vi "rec_manipJumpDAQreplicates_v02.vi"(0 "AI task in":refnum<k21>, 1 "number of samples":i32=-1, 3 "controls array in":refnum<vi>[](array[refnum]), 4 "AO task in":refnum<k21>, 5 "error in":errorcluster, 6 "Start Position":T1(ring), 7 "Jump On Time (s)":dbl, 8 "Use Current Position for Start Pos?":bool, 9 "Duration (s)":dbl, 10 "Jump Position":T1(ring), 11 "Jump Duration (s)":dbl, 12 "common cluster":T2) -> (14 "AI task out":refnum<k21>, 15 "data out (pA or mV)":waveform(dbl)(graph), 17 "control array out":refnum<vi>[](array[refnum]), 18 "AO task out":refnum<k21>, 19 "error out":errorcluster)   [LabVIEW 2019]
uses:
  multipatch/controls/multipatch_common_controls_v4.ctl
  machine_vision/controls/transform_cluster_actuator.ctl
  machine_vision/coordinate model vis/transform_properties_actuators.ctl
  pipette cleaning/pressure box/cleaning_soft/controls/actuator_cluster.ctl
  pipette cleaning/pressure box/cleaning_soft/controls/actuator_type.ctl
  pipette cleaning/pressure box/cleaning_soft/controls/pressure_box_control.ctl
  pipette cleaning/pressure box/cleaning_soft/controls/pressure_box_type.ctl
  controls/NH_method.ctl
  <vilib>/DAQmx/read.llb/DAQmx Read (Analog Wfm 1Chan NSamp).vi
  <vilib>/DAQmx/miscellaneous.llb/DAQmx Fill In Error Info.vi
  <resource>/objmgr/daqmx.rc
panel:
  out "AvailSampPerChan":u32
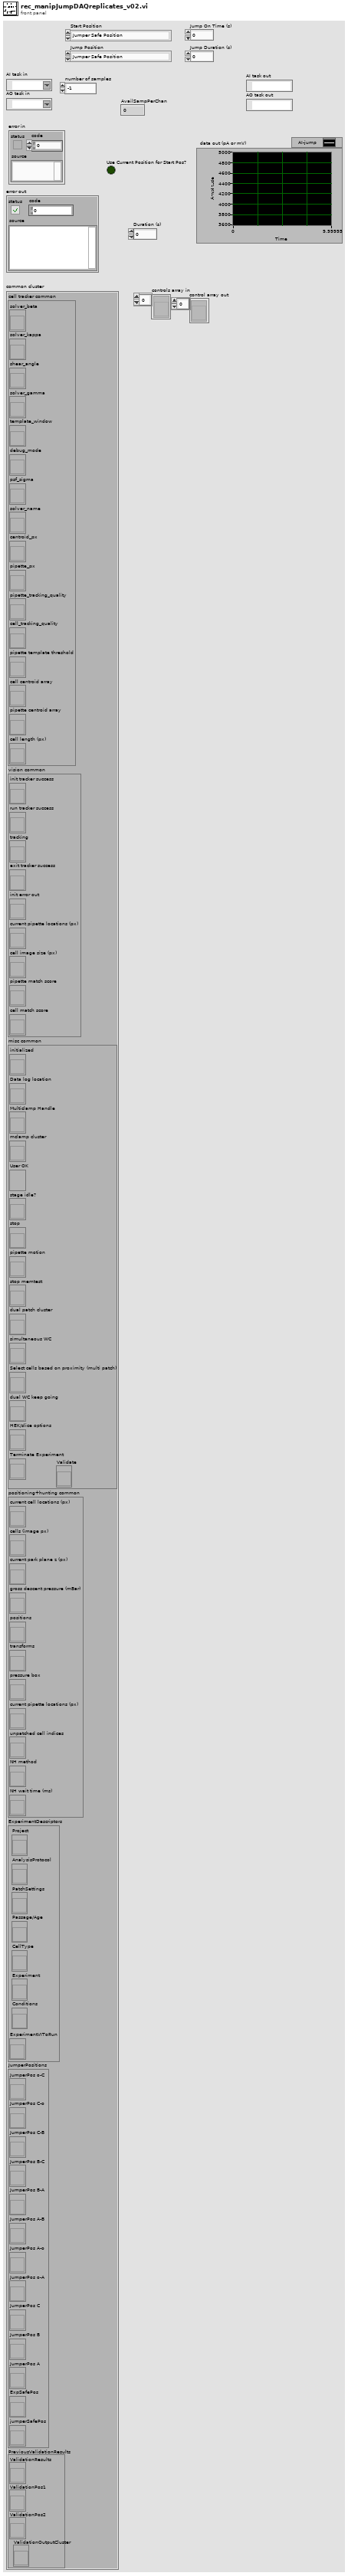
[diagram p1: front panel]
types:
  T1 = enum16{"Jumper Safe Position", "Experiment Safe Position", "Jumper Position A", "Jumper Position B", "Jumper Position C", "Jumper Position o-A", "Jumper Position A-o", "Jumper Position A-B", "Jumper Position B-A", "Jumper Position B-C", "Jumper Position C-B", "Jumper Position C-o", "Jumper Position o-C"}
  T2 = typedef "multipatch_common_controls_v4.ctl" = cluster{"cell tracker common":cluster{"solver_beta":refnum<vi>, "solver_kappa":refnum<vi>, "shear_angle":refnum<vi>, "solver_gamma":refnum<vi>, "template_window":refnum<vi>, "debug_mode":refnum<vi>, "psf_sigma":refnum<vi>, "solver_name":refnum<vi>, "centroid_px":refnum<vi>, "pipette_px":refnum<vi>, "pipette_tracking_quality":refnum<vi>, "cell_tracking_quality":refnum<vi>, "pipette template threshold":refnum<vi>, "cell centroid array":refnum<vi>, "pipette centroid array":refnum<vi>, "cell length (px)":refnum<vi>}, "vision common":cluster{"init tracker success":refnum<vi>, "run tracker success":refnum<vi>, "tracking":refnum<vi>, "exit tracker success":refnum<vi>, "init error out":refnum<vi>, "current pipette locations (px)":refnum<vi>, "cell image size (px)":refnum<vi>, "pipette match score":refnum<vi>, "cell match score":refnum<vi>}, "misc common":cluster{"initialized":refnum<vi>, "Data log location":refnum<vi>, "Multiclamp Handle":refnum<vi>, "mclamp cluster":refnum<vi>, "User OK":refnum<vi>, "stage idle?":refnum<vi>, "stop":refnum<vi>, "pipette motion":refnum<vi>, "stop memtest":refnum<vi>, "dual patch cluster":refnum<vi>, "simultaneous WC":refnum<vi>, "Select cells based on proximity (multi patch)":refnum<vi>, "dual WC keep going":refnum<vi>, "HEK/slice options":refnum<vi>, "Terminate Experiment":refnum<vi>, "Validate":refnum<vi>}, "positioning+hunting common":cluster{"current cell locations (px)":refnum<vi>, "cells (image px)":refnum<vi>, "current park plane z (px)":refnum<vi>, "gross descent pressure (mBar)":refnum<vi>, "positions":refnum<vi>, "transforms":refnum<vi>, "pressure box":refnum<vi>, "current pipette locations (px)":refnum<vi>, "unpatched cell indices":refnum<vi>, "NH method":refnum<vi>, "NH wait time (ms)":refnum<vi>}, "ExperimentDescriptors":cluster{"Project":refnum<vi>, "AnalysisProtocol":refnum<vi>, "PatchSettings":refnum<vi>, "Passage/Age":refnum<vi>, "CellType":refnum<vi>, "Experiment":refnum<vi>, "Conditions":refnum<vi>, "ExperimentVIToRun":refnum<vi>}, "JumperPositions":cluster{"JumperPos o-C":refnum<vi>, "JumperPos C-o":refnum<vi>, "JumperPos C-B":refnum<vi>, "JumperPos B-C":refnum<vi>, "JumperPos B-A":refnum<vi>, "JumperPos A-B":refnum<vi>, "JumperPos A-o":refnum<vi>, "JumperPos o-A":refnum<vi>, "JumperPos C":refnum<vi>, "JumperPos B":refnum<vi>, "JumperPos A":refnum<vi>, "ExpSafePos":refnum<vi>, "jumperSafePos":refnum<vi>}, "PreviousValidationResults":cluster{"ValidationResults":refnum<vi>, "ValidationPos1":refnum<vi>, "ValidationPos2":refnum<vi>, "ValidationOutputCluster":refnum<vi>}}
  T3 = enum16{"manipulator 1", "manipulator 2", "manipulator 3", "manipulator 4"}
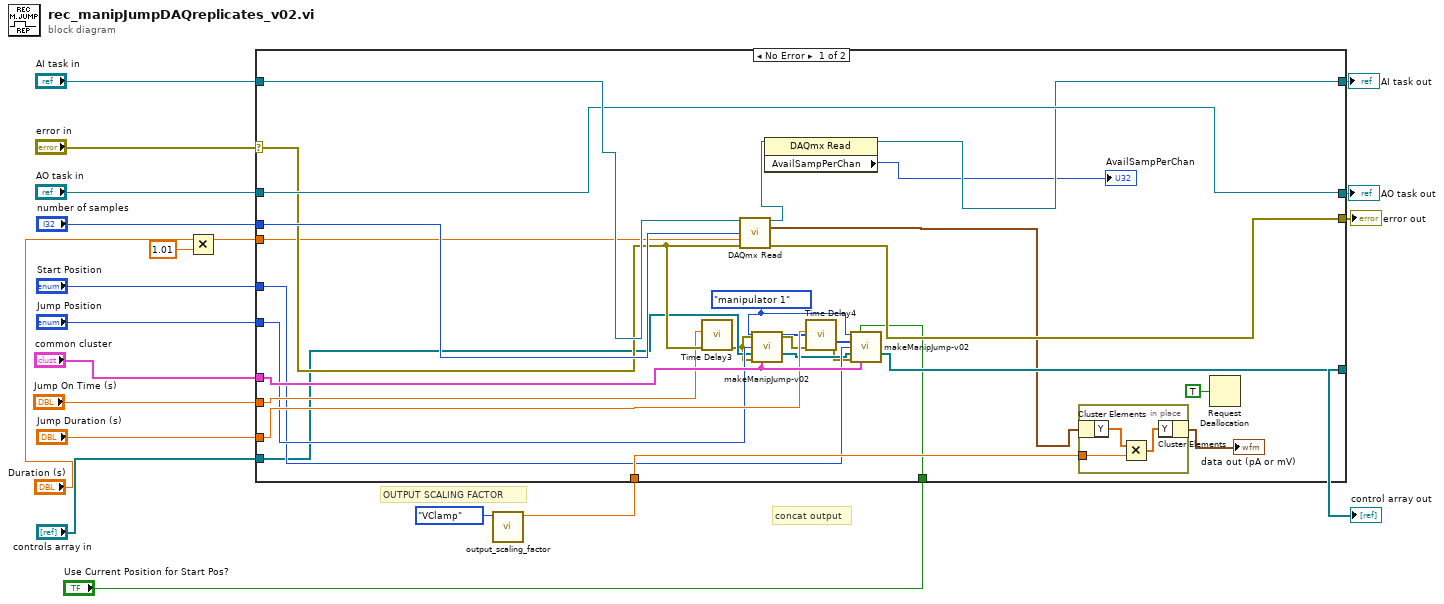
[diagram p0: block diagram]
diagram:
  # "concat output"
  # "OUTPUT SCALING FACTOR"
  n1 = Multiply(x="Duration (s)", y=1.01) -> (x*y=w3:dbl)
  n2 = call "output_scaling_factor.vi"("which clamp"=enum16{"VClamp", "IClamp"}."VClamp") -> ("output scaling factor"=w14:dbl)  [unwired: 10 in]
  n3 = case shown="No Error" "error in" {
    selector: "error in" -> [w41 w51]
    tunnel: "AI task in" -> [w45 w53]
    tunnel: "AO task in" -> [w43 w52]
    tunnel: [w43 w52] -> w17
    tunnel: [w33 w53] -> w16
    tunnel: [w44 w51] -> w15
    tunnel: w14 -> [w46 _]
    tunnel: "number of samples" -> [w42 _]
    tunnel: "common cluster" -> [w40 _]
    tunnel: "Jump On Time (s)" -> [w39 _]
    tunnel: "Jump Duration (s)" -> [w38 _]
    tunnel: "Start Position" -> [w36 _]
    tunnel: "Jump Position" -> [w37 _]
    tunnel: "controls array in" -> [w35 w50]
    tunnel: [w34 w50] -> w5
    tunnel: w3 -> [w31 _]
    tunnel: "Use Current Position for Start Pos?" -> [w30 _]
    frame No Error {
      w28 = T3."manipulator 1" ("which manipulator")
      n4 = call "Time Delay3"("error in (no error)"=w41, "Delay Time (s)"=w39) -> ("error out"=w24:errorcluster)  [unwired: 9 in]
      n5 = call-poly <vilib>:"DAQmx Read.vi"("task/channels in"=w45, "number of samples per channel"=w42, "timeout"=w31, "error in"=w41) -> ("task out"=w26:refnum<k21>, "data"=w22:waveform(dbl), "error out"=w44:errorcluster)  [unwired: 9 in]
      n6 = call "makeManipJump-v02.vi"("which manipulator"=w28, "Which Jumper Position to move to?"=w37, "controls array in"=w35, "error in"=w24, "common cluster"=w40) -> ("currentPos"=w23:i32[], "control array out"=w27:refnum<vi>[])  [unwired: 8 in, 1 out]
      n7 = property class="DAQmx Read"(reference=w26) -> (reference out=w33:refnum<k21>, "AvailSampPerChan"=→"AvailSampPerChan":u32)  [unwired: 1 in, 1 out]
      n8 = call "Time Delay4"("error in (no error)"=w24, "Delay Time (s)"=w38) -> ("error out"=w25:errorcluster)  [unwired: 9 in]
      n9 = call "makeManipJump-v02.vi"("which manipulator"=w28, "Use Current Position for Start Pos?"=w30, "Orig Pos"=w23, "Which Jumper Position to move to?"=w36, "controls array in"=w27, "error in"=w25, "common cluster"=w40) -> ("control array out"=w34:refnum<vi>[])  [unwired: 6 in, 2 out]
      n10 = in-place {
        in-place-border: w46 -> [w49]
        n11 = in-place-cluster #1(w22) -> ("Y"=w47:dbl[])
        n12 = Multiply(x=w47, y=w49) -> (x*y=w48:dbl[])
        n13 = in-place-cluster #1("Y"=w48) -> (→"data out (pA or mV)":waveform(dbl))
      }
      n14 = Request Deallocation(TRUE ("flag")) -> ()
    }
    frame Error {
    }
  }
  "AI task out" <- w16
  "AO task out" <- w17
  "error out" <- w15
  "control array out" <- w5
